vi "Shooter and Intake.vi"() -> ()   [LabVIEW 2012]
uses:
  Globals/Jaguar Commands.vi
  Globals/Robot Build.vi
  <vilib>/Rock Robotics/WPI/Joystick/WPI_JoystickGetSetRefNum.vi
  Globals/Shooter Gathering Velocity.vi
  Globals/Shooter Testing.vi
  Globals/Calculated Shooter Speed.vi
panel:
  in  "Uber Speed":dbl=12500.0
  in  "Fender Speed":dbl=5800.0
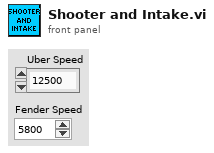
[diagram p1: front panel]
types:
  T1 = typedef "WPI_JoystickDevRef.ctl" = cluster{"Device":T2}
  T2 = typedef "WPI_JoystickDeviceEnum.ctl" = enum16{"USB 1", "USB 2", "USB 3", "USB 4", "Kinect 1", "Kinect 2"}
  T3 = typedef "WPI_JoystickButtonState.ctl" = cluster{"Button 1":bool, "Button 2":bool, "Button 3":bool, "Button 4":bool, "Button 5":bool, "Button 6":bool, "Button 7":bool, "Button 8":bool, "Button 9":bool, "Button 10":bool, "Button 11":bool, "Button 12":bool}
  T4 = cluster{"axis 1 (x)":dbl, "axis 2 (y)":dbl, "axis 3 (throttle)":dbl, "axis 4":dbl, "axis 5":dbl, "axis 6":dbl}
  T5 = typedef "Robot Build.ctl" = enum16{"Practice Bot", "Competition Bot"}
  T6 = typedef "WPI_MotorControlDeviceRef.ctl" = cluster{"DeviceStatus":errorcluster, "Type":enum16{"PWM", "CAN"}, "PWM":cluster{"Digital Module":T7, "PWM Channel":T8, "DeadBand":T9}, "CAN":cluster{"Device Number":u8, "Control Mode":T10, "Semaphore":T11, "Max Vout":dbl}, "Invert":bool, "TransformRef":T12, "InvTransformRef":T12}
  T7 = typedef "FPGA_TypedefDigitalModule.ctl" = enum16{"Digital Module 1", "Digital Module 2"}
  T8 = typedef "FPGA_DIOPWMChannel.ctl" = enum8{"PWM 1", "PWM 2", "PWM 3", "PWM 4", "PWM 5", "PWM 6", "PWM 7", "PWM 8", "PWM 9", "PWM 10", "Invalid"}
  T9 = typedef "WPI_PWMDeadband.ctl" = cluster{"Name":string, "maxPositivePwm":i32, "minPositivePwm":i32, "centerPwm":i32, "maxNegativePwm":i32, "minNegativePwm":i32, "angularRange":u16}
  T10 = typedef "WPI_CANJaguar_ControlMode.ctl" = enum8{"Percent VBus", "Current", "Speed", "Position", "Voltage"}
  T11 = typedef "Semaphore RefNum" = refnum<k1>
  T12 = typedef "WPI_PWMTransform_ConPane.ctl" = refnum<vi>
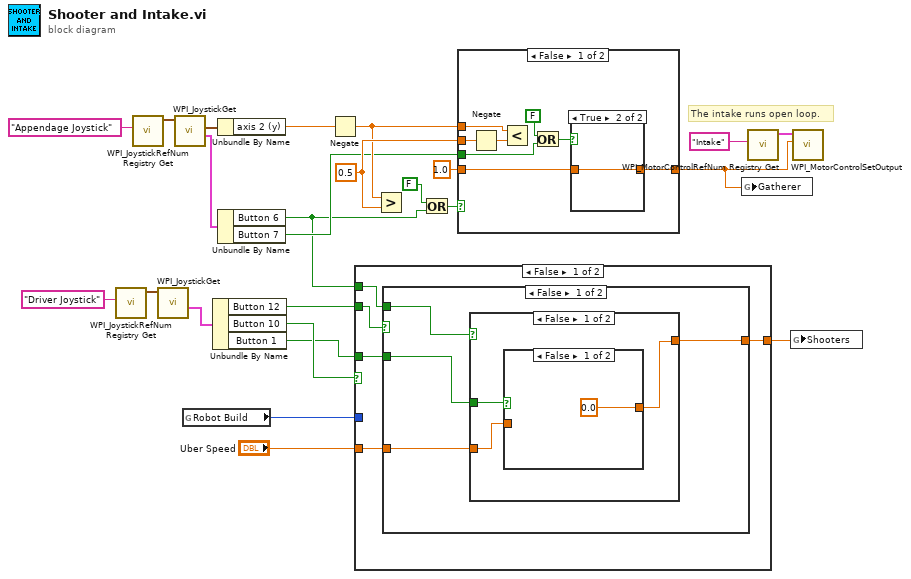
[diagram p0: block diagram]
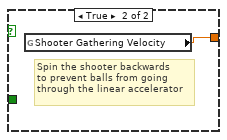
[diagram p3: hidden frame]
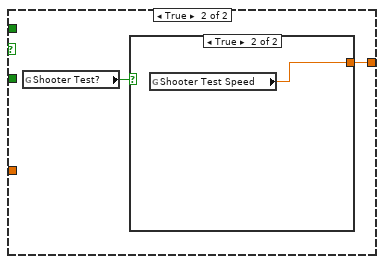
[diagram p4: hidden frame]
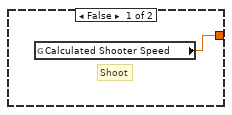
[diagram p5: hidden frame]
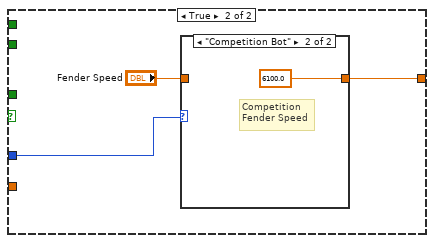
[diagram p6: hidden frame]
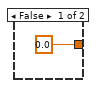
[diagram p8: hidden frame]
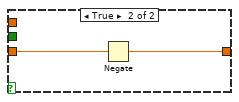
[diagram p9: hidden frame]
diagram:
  w17 = 0.5 ("y")
  # "The intake runs open loop."
  n1 = call <vilib>:"WPI_JoystickRefNum Registry Get.vi"("refnum name"="Driver Joystick") -> ("JoystickDevRef"=w12:T1)  [unwired: 9 in, 1 out]
  n2 = call <vilib>:"WPI_JoystickRefNum Registry Get.vi"("refnum name"="Appendage Joystick") -> ("JoystickDevRef"=w21:T1)  [unwired: 9 in, 1 out]
  n3 = call <vilib>:"WPI_JoystickGet.vi"("JoystickDevRef"=w12) -> ("Buttons"=w11:T3)  [unwired: 4 in, 2 out]
  n4 = call <vilib>:"WPI_JoystickGet.vi"("JoystickDevRef"=w21) -> ("Buttons"=w24:T3, "Axes"=w22:T4)  [unwired: 4 in, 1 out]
  n5 = global read "Robot Build.vi" "Robot Build"() -> (w4:T5)
  n6 = Unbundle By Name(w11) -> ("Button 12"=w10:bool, "Button 10"=w6:bool, "Button 1"=w2:bool)
  n7 = Unbundle By Name(w22) -> ("axis 2 (y)"=w23:dbl)
  n8 = Unbundle By Name(w24) -> ("Button 6"=w5:bool, "Button 7"=w8:bool)
  n9 = Negate(x=w23) -> (-x=w16:dbl)
  n10 = case shown="False" w6 {
    tunnel: w10 -> [w29 _]
    tunnel: [w28 w46] -> w9
    tunnel: w5 -> [w27 _]
    tunnel: w4 -> [_ w44]
    tunnel: "Uber Speed" -> [w26 _]
    tunnel: w2 -> [w25 _]
    frame False {
      n11 = case shown="False" w29 {
        tunnel: [w33 w41] -> w28
        tunnel: w27 -> [w32 _]
        tunnel: w26 -> [w31 _]
        tunnel: w25 -> [w30 _]
        frame False {
          n12 = case shown="False" w32 {
            tunnel: [w36 w39] -> w33
            tunnel: w31 -> [w35 _]
            tunnel: w30 -> [w34 _]
            frame False {
              n13 = case shown="False" w34 {
                tunnel: [0.0 w38] -> w36
                tunnel: w35 -> [_ w38]
                frame False {
                }
                frame True {
                }
              }
            }
            frame True {
              # "Spin the shooter backwards\nto prevent balls from going\nthrough the linear accelerator"
              n14 = global read "Shooter Gathering Velocity.vi" "Shooter Gathering Velocity"() -> (w39:dbl)
            }
          }
        }
        frame True {
          n15 = global read "Shooter Testing.vi" "Shooter Test?"() -> (w40:bool)
          n16 = case shown="True" w40 {
            tunnel: [w42 w43] -> w41
            frame False {
              # "Shoot"
              n17 = global read "Calculated Shooter Speed.vi" "Calculated Shooter Speed"() -> (w42:dbl)
            }
            frame True {
              n18 = global read "Shooter Testing.vi" "Shooter Test Speed"() -> (w43:dbl)
            }
          }
        }
      }
    }
    frame True {
      n19 = case shown="\"Competition Bot\"" w44 {
        tunnel: [w47 6100.0 ("Fender Speed")] -> w46
        tunnel: "Fender Speed" -> [w47 _]
        frame "Practice Bot", Default {
        }
        frame "Competition Bot" {
          # "Competition\nFender Speed"
        }
      }
    }
  }
  n20 = Greater?(x=w16, y=w17) -> ()  [unwired: 1 out]
  n21 = Or(x=FALSE, y=w5) -> (x .or. y?=w14:bool)
  n22 = case shown="False" w14 {
    tunnel: 1.0 ("Percent VBus") -> [w53 w60]
    tunnel: [w52 w59] -> w7
    tunnel: w17 -> [w56 _]
    tunnel: w16 -> [w54 _]
    tunnel: w8 -> [w51 _]
    frame False {
      n23 = Negate(x=w56) -> (-x=w55:dbl)
      n24 = Less?(x=w54, y=w55) -> ()  [unwired: 1 out]
      n25 = Or(x=FALSE, y=w51) -> (x .or. y?=w50:bool)
      n26 = case shown="True" w50 {
        tunnel: w53 -> [_ w58]
        tunnel: [0.0 w58] -> w52
        frame False {
        }
        frame True {
        }
      }
    }
    frame True {
      n27 = Negate(x=w60) -> (-x=w59:dbl)
    }
  }
  n28 = global write "Jaguar Commands.vi" "Gatherer"(w7) -> ()
  n29 = call <vilib>:"WPI_MotorControlRefNum Registry Get.vi"("refnum name"="Intake") -> ("MotorControlDevRef"=w18:T6)  [unwired: 9 in, 1 out]
  n30 = global write "Jaguar Commands.vi" "Shooters"(w9) -> ()
  n31 = call <vilib>:"WPI_MotorControlSetOutput.vi"("Output"=w7, "MotorControlDevRef"=w18) -> ()  [unwired: 7 in, 3 out]
